vi "Draw Axes at Point.vi"(5 "Thickness (Default: 1)":i32=1, 6 "Camera Parameters":T1, 7 "Length":dbl=1.0, 8 "error in (no error)":errorcluster, 9 "Point (Default 0,0,0)":T7, 10 "Pose":T4, 11 "ARGB Image in":T8) -> (0 "error out":errorcluster, 3 "ARGB Image (Duplicate)":T8)   [LabVIEW 2020, in "ar.lvlib"]
uses:
  ar.lvlib
  image/ARGB Image.ctl
  common/Object Point (Float).ctl
  Pose.ctl
  rvec.ctl
  tvec.ctl
  common/Camera Parameters.ctl
  common/Camera Matrix.ctl
  common/Camera Distortion Coefficients.ctl
  common/Image Point (Integer).ctl
  image/ARGB Colour.ctl
  image/Draw Line (ARGB).vi
  03c70bae-05f7-4e6e-967f-c3ec9382dd74.vi
  image/ARGB Colour to U32 Pixel Value.vi
  image/Draw Line (ARGB).vi/85aa1280-0fac-47da-ba54-33850455c996.vi
  common/Module Path.vi
  <vilib>/Utility/error.llb/Error Cluster From Error Code.vi
  image/image.lvlib
  common/common.lvlib
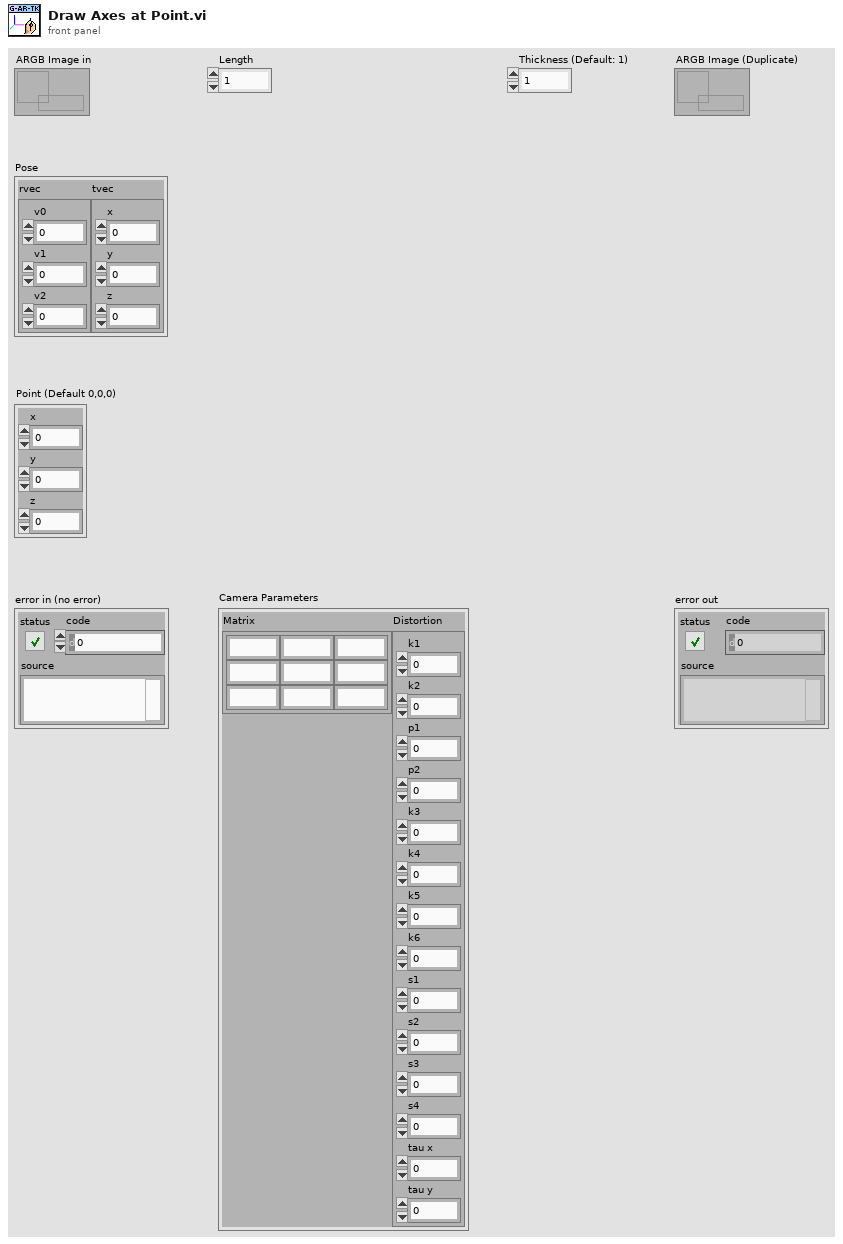
[diagram p1: front panel]
types:
  T1 = typedef "common.lvlib/Camera Parameters.ctl" = cluster{"Matrix":T2, "Distortion":T3}
  T2 = typedef "common.lvlib/Camera Matrix.ctl" = cluster{"m 0,0":dbl, "m 0,1":dbl, "m 0,2":dbl, "m 1,0":dbl, "m 1,1":dbl, "m 1,2":dbl, "m 2,0":dbl, "m 2,1":dbl, "m 2,2":dbl}
  T3 = typedef "common.lvlib/Camera Distortion Coefficients.ctl" = cluster{"k1":dbl, "k2":dbl, "p1":dbl, "p2":dbl, "k3":dbl, "k4":dbl, "k5":dbl, "k6":dbl, "s1":dbl, "s2":dbl, "s3":dbl, "s4":dbl, "tau x":dbl, "tau y":dbl}
  T4 = typedef "ar.lvlib/Pose.ctl" = cluster{"rvec":T5, "tvec":T6}
  T5 = typedef "ar.lvlib/rvec.ctl" = cluster{"v0":dbl, "v1":dbl, "v2":dbl}
  T6 = typedef "ar.lvlib/tvec.ctl" = cluster{"x":dbl, "y":dbl, "z":dbl}
  T7 = typedef "common.lvlib/Object Point (Float).ctl" = cluster{"x":dbl, "y":dbl, "z":dbl}
  T8 = typedef "image.lvlib/ARGB Image.ctl" = refnum<data-value>
  T9 = typedef "common.lvlib/Image Point (Integer).ctl" = cluster{"x":i32, "y":i32}
  T10 = typedef "common.lvlib/Image Point (Float).ctl" = cluster{"x":dbl, "y":dbl}
  T11 = typedef "image.lvlib/ARGB Colour.ctl" = cluster{"Alpha":u8, "RGB":u32}
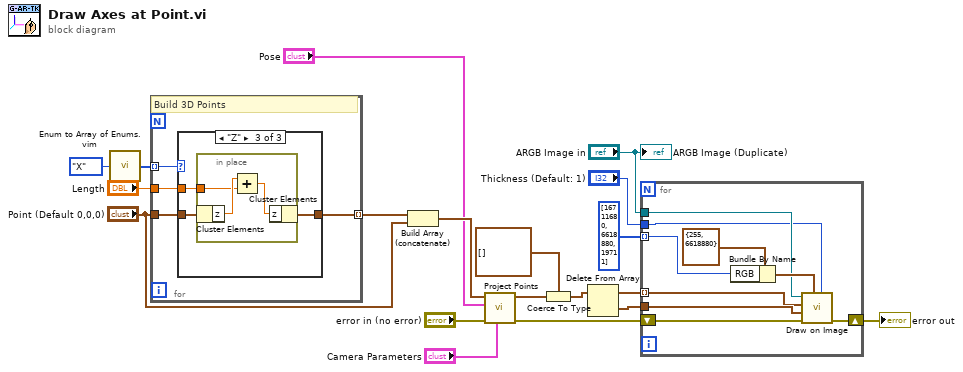
[diagram p0: block diagram]
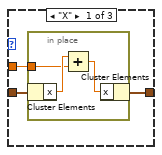
[diagram p2: hidden frame]
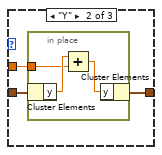
[diagram p3: hidden frame]
diagram:
  n1 = call "Enum to Array of Enums.vim"("enum"=enum16{"X", "Y", "Z"}."X") -> ("array of enums"=w17:enum16{"X", "Y", "Z"}[])
  n2 = for {
    tunnel: "Point (Default 0,0,0)" -> [w22]
    tunnel: w17 -> [w23] mode=indexing
    tunnel: "Length" -> [w21]
    tunnel: [w20] -> w15 mode=indexing
    # "Build 3D Points"
    n3 = case shown="\"Z\"" w23 {
      tunnel: w22 -> [w26 w32 w38]
      tunnel: w21 -> [w25 w31 w37]
      tunnel: [w24 w30 w36] -> w20
      frame "X" {
        n4 = in-place {
          in-place-border: w25 -> [w28]
          n5 = in-place-cluster #1(w26) -> ("x"=w29:dbl)
          n6 = Add(x=w29, y=w28) -> (x+y=w27:dbl)
          n7 = in-place-cluster #1("x"=w27) -> (w24:T7)
        }
      }
      frame "Y" {
        n8 = in-place {
          in-place-border: w31 -> [w34]
          n9 = in-place-cluster #2(w32) -> ("y"=w35:dbl)
          n10 = Add(x=w35, y=w34) -> (x+y=w33:dbl)
          n11 = in-place-cluster #2("y"=w33) -> (w30:T7)
        }
      }
      frame "Z" {
        n12 = in-place {
          in-place-border: w37 -> [w40]
          n13 = in-place-cluster #3(w38) -> ("z"=w41:dbl)
          n14 = Add(x=w41, y=w40) -> (x+y=w39:dbl)
          n15 = in-place-cluster #3("z"=w39) -> (w36:T7)
        }
      }
    }
  }
  n16 = Build Array (concatenate)(w15, "Point (Default 0,0,0)") -> (w12:T7[])
  n17 = call "Project Points.vi"("Camera Parameters"="Camera Parameters", "error in (no error)"="error in (no error)", "Pose"="Pose", "Object Points"=w12) -> ("error out"=w7:errorcluster, "Image Points"=w9:T10[])  [unwired: 6 in]
  n18 = Coerce To Type(0:w9, 1:T9[] [] ("Array")) -> (2:w2:T9[])
  n19 = Delete From Array(array=w2) -> (deleted portion=w19:T9, array with subset deleted=w8:T9[])  [unwired: 2 in]
  n20 = for {
    shift-right: [w50] -> w5
    shift-left: w7 -> [w49]
    tunnel: w19 -> [w45]
    tunnel: w8 -> [w42] mode=indexing
    tunnel: u32[] [16711680, 6618880, 19711] ("RGB") -> [w46] mode=indexing
    tunnel: "ARGB Image in" -> [w44]
    tunnel: "Thickness (Default: 1)" -> [w43]
    n21 = Bundle By Name(cluster=T11 {"Alpha"=255, "RGB"=6618880} ("ARGB Colour"), "RGB"=w46) -> (w47:T11)
    n22 = call-poly "Draw on Image.vi"("Thickness (Default: 1)"=w43, "ARGB Colour"=w47, "error in (no error)"=w49, "Point B"=w45, "Point A"=w42, "ARGB Image"=w44) -> ("error out"=w50:errorcluster)  [unwired: 4 in, 1 out]
  }
  "error out" <- w5
  "ARGB Image (Duplicate)" <- "ARGB Image in"
